vi "Convert Font Style.vi"(1 "Font Style In":T1) -> (0 "Font Style Out":i32)   [LabVIEW 2020, in "Dot Net UI Controls.lvlib"]
uses:
  Dot Net UI Controls.lvlib
  Font Style.ctl
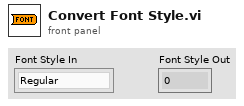
[diagram p1: front panel]
types:
  T1 = typedef "Dot Net UI Controls.lvlib/Font Style.ctl" = enum16{"Regular", "Bold", "Italic", "Underline", "Strikeout"}
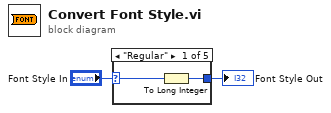
[diagram p0: block diagram]
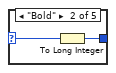
[diagram p2: hidden frame]
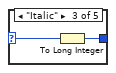
[diagram p3: hidden frame]
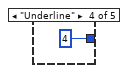
[diagram p4: hidden frame]
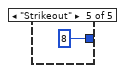
[diagram p5: hidden frame]
diagram:
  n1 = case shown="\"Regular\"" "Font Style In" {
    selector: "Font Style In" -> [w4 w6 w8 _ _]
    tunnel: [w3 w5 w7 4 8] -> w2
    frame "Regular" {
      n2 = To Long Integer(number=w4) -> (32bit integer=w3:i32)
    }
    frame "Bold" {
      n3 = To Long Integer(number=w6) -> (32bit integer=w5:i32)
    }
    frame "Italic" {
      n4 = To Long Integer(number=w8) -> (32bit integer=w7:i32)
    }
    frame "Underline" {
    }
    frame "Strikeout" {
    }
  }
  "Font Style Out" <- w2
